vi "AD Convertor linear fit.vi"() -> ()   [LabVIEW 2015]
uses:
  <vilib>/Analysis/NI_AALPro.lvlib
panel:
  out "INTERCEPT":ext format="%.2f"
  out "SLOPE":ext format="%.2f"
  out "?":cluster{ext, ext}[](graph)
  in  "?":ext[][](array[numeric])=[[0.0, 0.49], [20.0, 7.52], [40.0, 15.79], [80.0, 32.279999999999999999], [100.0, 38.330000000000000002], [200.0, 77.64], [0.0, 0.49], [0.0, 0.49], [0.0, 0.49]] format="%.2f"
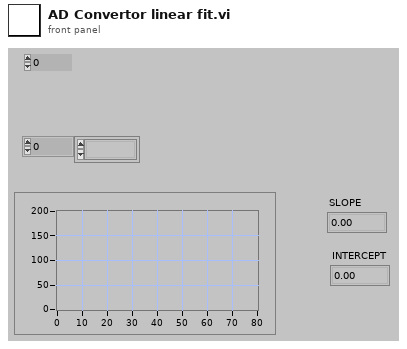
[diagram p1: front panel]
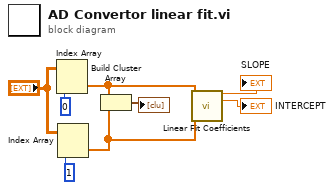
[diagram p0: block diagram]
diagram:
  n1 = Index Array(array="?", index (col)=0) -> (element=w4:ext[])  [unwired: 1 in]
  n2 = Index Array(array="?", index (col)=1) -> (element=w3:ext[])  [unwired: 1 in]
  n3 = Build Cluster Array(w3, w4) -> (→"?":cluster{ext, ext}[])
  n4 = call <vilib>:"Linear Fit Coefficients.vi"("Y"=w4, "X"=w3) -> ("slope"=→"SLOPE":dbl, "intercept"=→"INTERCEPT":dbl)  [unwired: 11 in, 1 out]
